vi "Calc_Remaining_Time.vi"(2 "Currently on Row":i32, 3 "Table In":T1[](array[typedef]) {"Row Duration (mins)" format="%#.1f"; "Row No" min=0; "Trace Gas Concentration (%)" min=0.0 format="%#.2f"; "Emission Rate (l/min)" format="%#.2f"; "Tunnel Speed" format="%#.2f"; "Start X" format="%#.2f"; "Start Y" format="%#.2f"; "Start Z" format="%#.2f"; "End X" format="%#.2f"; "End Y" format="%#.2f"; "End Z" format="%#.2f"; "Averaging time (min)" min=0.0 format="%#.2f"}) -> (0 "Estimated Completion time":string, 1 "Table Out":T1[](array[typedef]) {"Row Duration (mins)" format="%#.1f"; "Row No" min=0; "Trace Gas Concentration (%)" min=0.0 format="%#.2f"; "Emission Rate (l/min)" format="%#.2f"; "Tunnel Speed" format="%#.2f"; "Start X" format="%#.2f"; "Start Y" format="%#.2f"; "Start Z" format="%#.2f"; "End X" format="%#.2f"; "End Y" format="%#.2f"; "End Z" format="%#.2f"; "Averaging time (min)" min=0.0 format="%#.2f"})   [LabVIEW 2010]
uses:
  Traverse_cluster.ctl
  Spacing.ctl
  Controls/Multi_run_mode.ctl
  Controls/Overhead.ctl
  Globals/Extra_Commands_Global.vi
  Globals/Trav_pos_global.vi
panel:
  # "X           Y            Z"
  # "Start"
  # "End"
  # "X           Y            Z"
  # "Start"
  # "End"
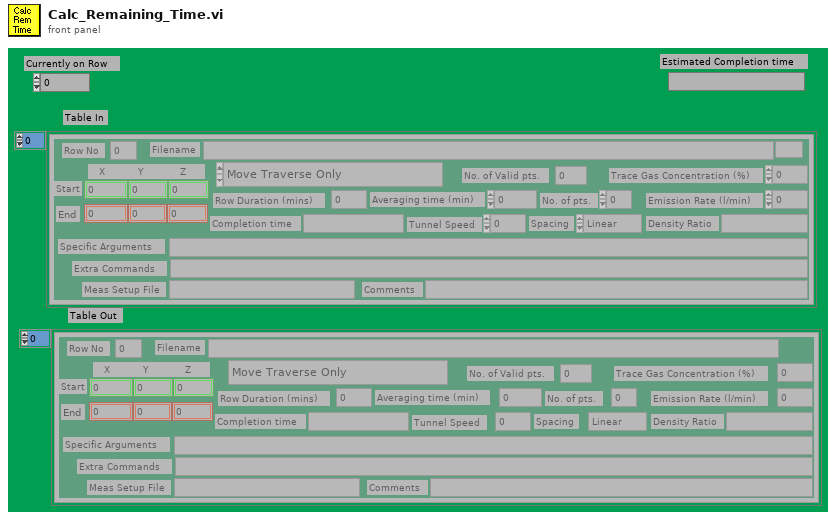
[diagram p1: front panel]
types:
  T1 = typedef "Traverse_cluster.ctl" = cluster{"Start X":dbl, "Start Y":dbl, "Start Z":dbl, "End X":dbl, "End Y":dbl, "End Z":dbl, "No. of pts.":i32, "Spacing":T2, "Filename":path, "Tunnel Speed":dbl, "Averaging time (min)":dbl, "Extra Commands":string, "Specific Arguments":string, "Emission Rate (l/min)":dbl, "Trace Gas Concentration (%)":dbl, "Density Ratio":string, "Comments":string, "Row No":i32, "Row Type Selector":T3, "Completion time":string, "Row Duration (mins)":dbl, "No. of Valid pts.":i32, "Meas Setup File":string}
  T2 = typedef "Spacing.ctl" = enum16{"Linear", "Log", "Gauss", "Specified", "N/A"}
  T3 = typedef "Multi_run_mode.ctl" = enum16{"Move Traverse Only", "Set Tunnel Speed Only", "Set Source Only", "Set Measurement Conditions", "Single Measurement", "Vertical Profile", "Lateral Profile", "Longitudinal Profile", "Explore Volume", "Multi-Axis Profile", "Auto Calibrate", "Meas Fast FID Bkgnd", "Check Beam Power", "Scanning Valve Measurement", "Run VI Named:", "Set ADAM Ch", "Wait (minutes)", "Send Message", "Synchronize With:", "Fall Back to this Row", "Turn Off Row Repeating", "Blank Row"}
  T4 = typedef "Overhead.ctl" = enum16{"Update total times", "Read Current Overhead", "Re Scale totals to 3 hrs", "Initialise totals to 3hr"}
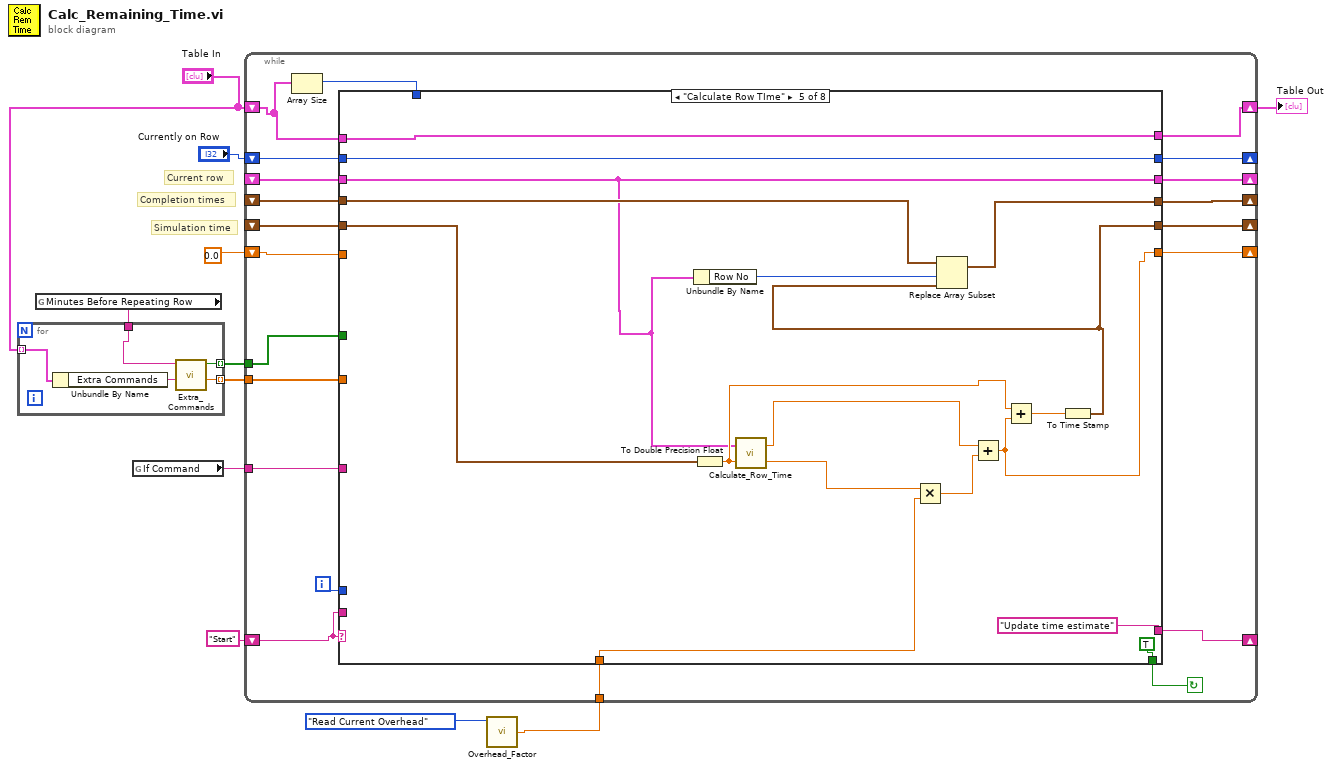
[diagram p0: block diagram]
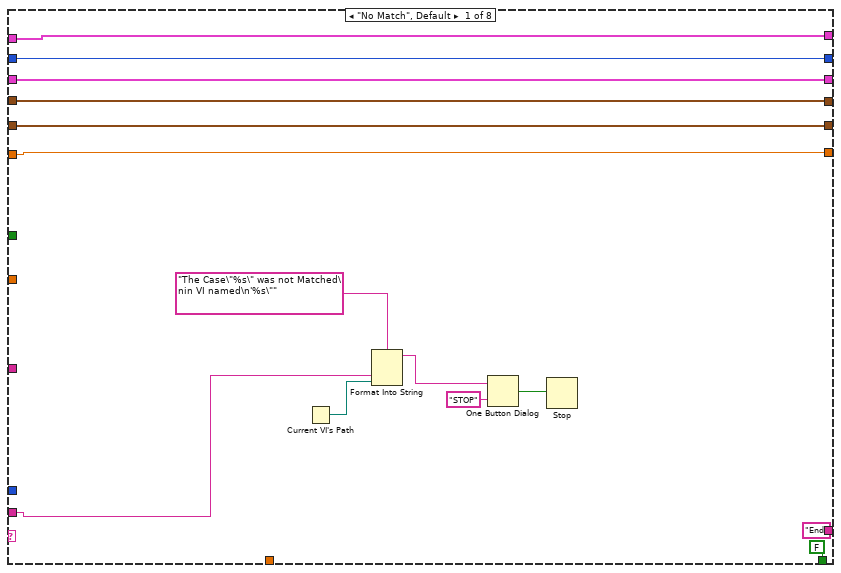
[diagram p2: hidden frame]
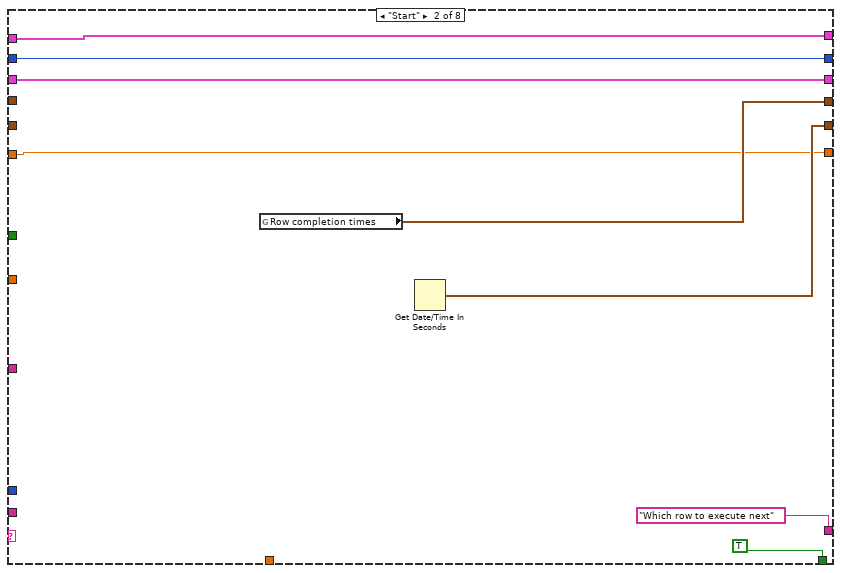
[diagram p3: hidden frame]
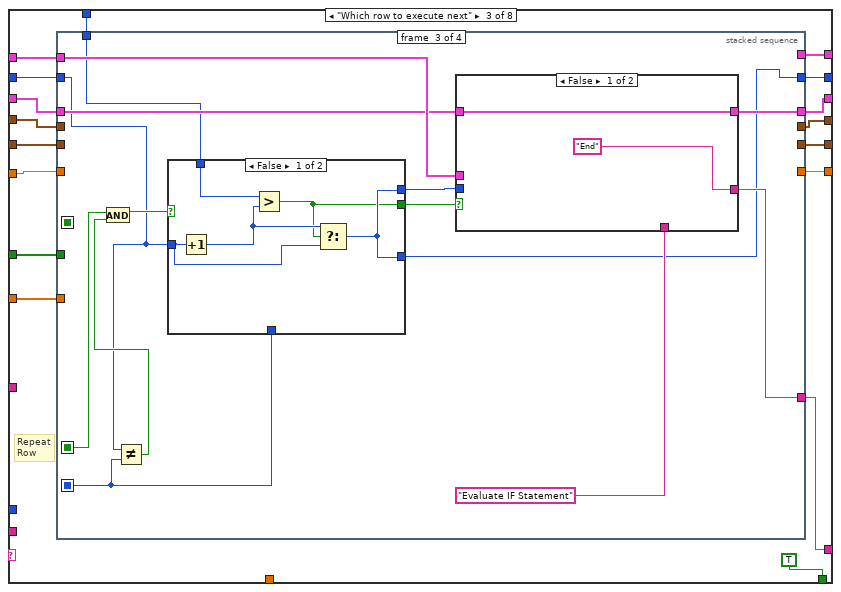
[diagram p4: hidden frame]
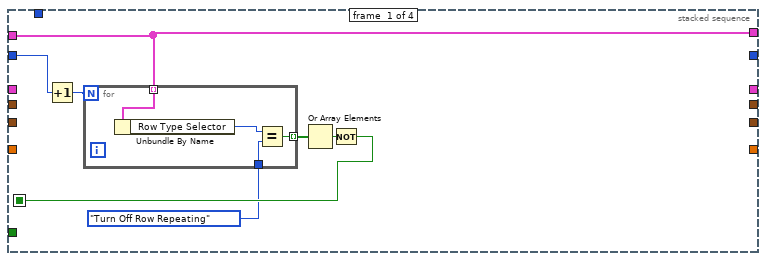
[diagram p5: hidden frame]
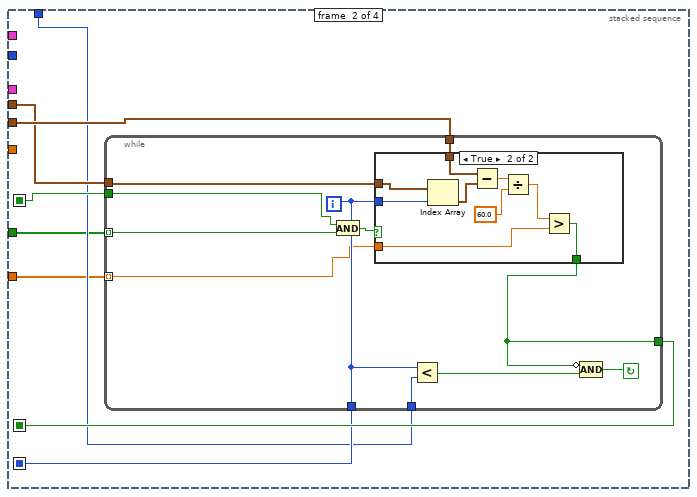
[diagram p6: hidden frame]
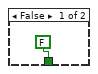
[diagram p7: hidden frame]
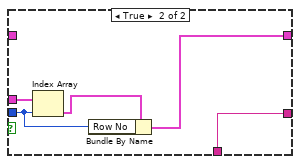
[diagram p8: hidden frame]
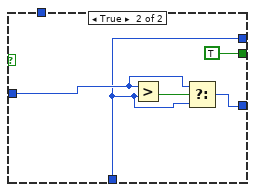
[diagram p9: hidden frame]
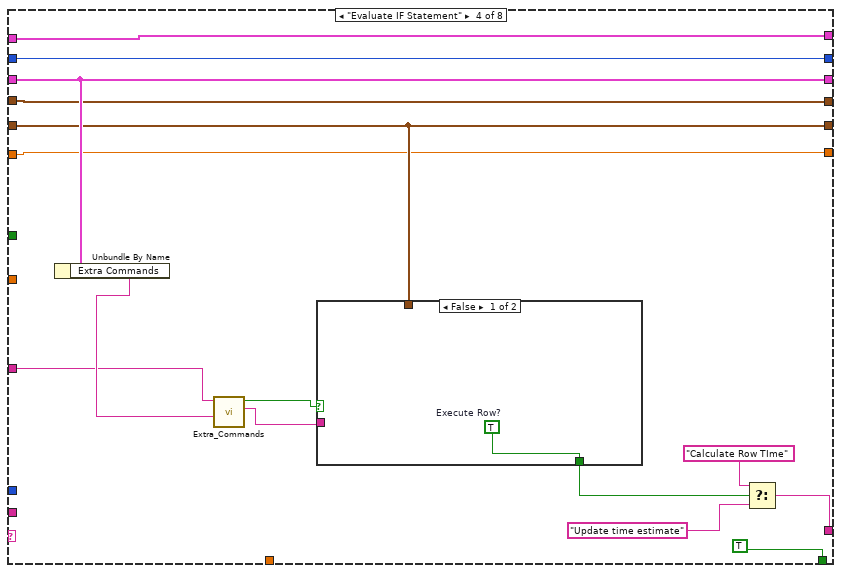
[diagram p11: hidden frame]
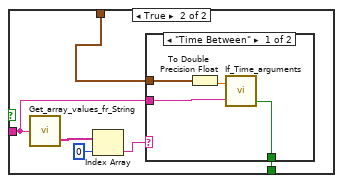
[diagram p12: hidden frame]
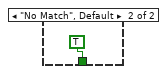
[diagram p13: hidden frame]
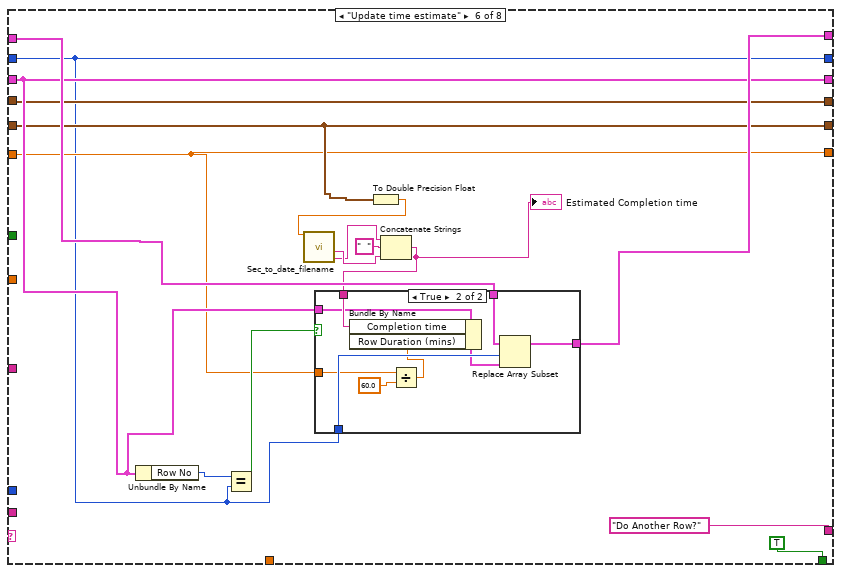
[diagram p14: hidden frame]
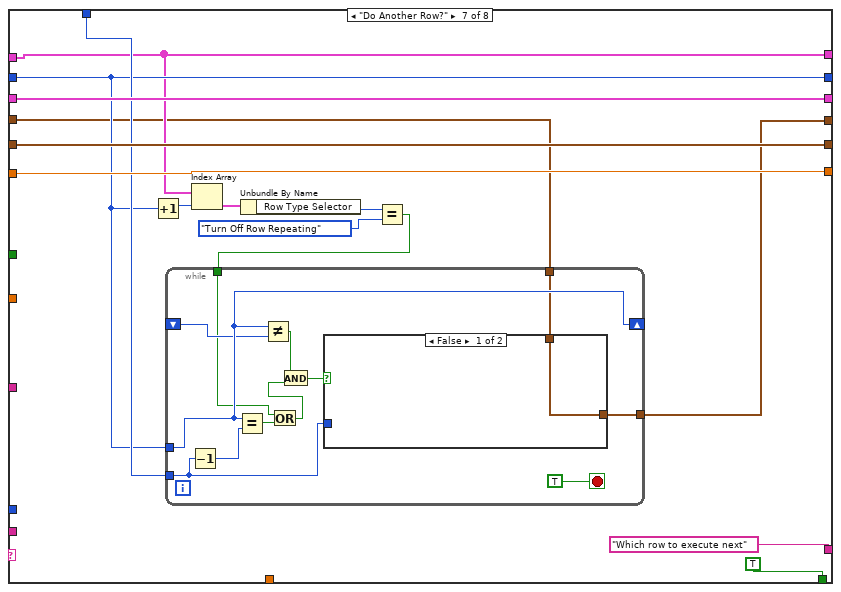
[diagram p16: hidden frame]
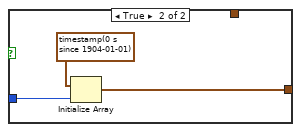
[diagram p17: hidden frame]
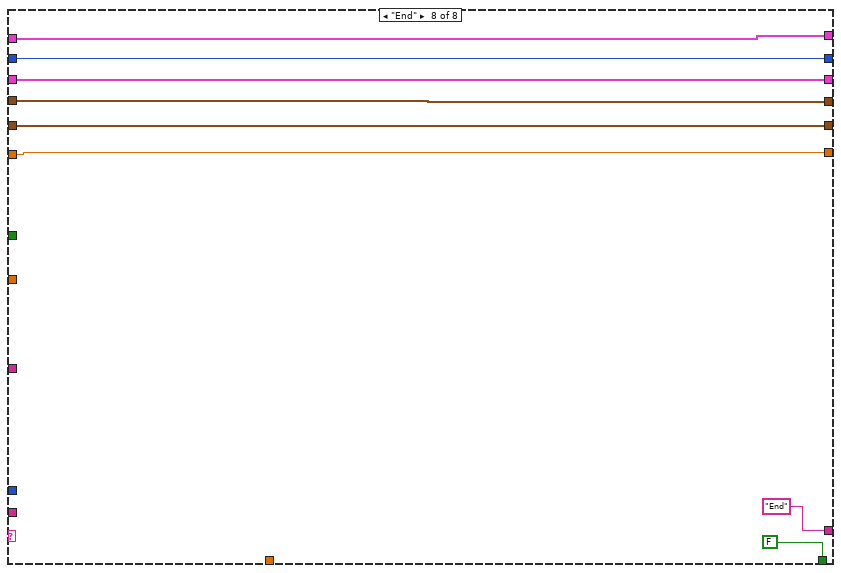
[diagram p18: hidden frame]
diagram:
  # "Simulation time"
  # "Completion times"
  # "Current row"
  n1 = global read "Extra_Commands_Global.vi" "Minutes Before Repeating Row"() -> (w1:string)
  n2 = for {
    tunnel: "Table In" -> [w15] mode=indexing
    tunnel: [w14] -> w3 mode=indexing
    tunnel: [w13] -> w2 mode=indexing
    tunnel: w1 -> [w12]
    n3 = Unbundle By Name(w15) -> ("Extra Commands"=w16:string)
    n4 = call "Extra_Commands.vi"("String to Search"=w16, "Command"=w12) -> ("Numeric Value"=w13:dbl, "Command Found"=w14:bool)  [unwired: 1 in, 3 out]
  }
  n5 = global read "Extra_Commands_Global.vi" "If Command"() -> (w7:string)
  n6 = call "Overhead_Factor.vi"("Mode"=Overhead."Read Current Overhead") -> ("Current Overhead Factor"=w8:dbl)  [unwired: 3 in]
  n7 = while {
    shift-left: "Start" -> [w35]
    shift-right: [w34] -> _
    shift-right: [w32] -> w10
    shift-left: "Table In" -> [w21]
    tunnel: w8 -> [w31]
    shift-right: [w30] -> _
    shift-left: _ -> [w29]
    shift-right: [w25] -> _
    shift-left: _ -> [w26]
    shift-right: [w27] -> _
    shift-left: _ -> [w28]
    shift-right: [w22] -> _
    shift-left: "Currently on Row" -> [w23]
    tunnel: w7 -> [w24]
    shift-right: [w20] -> _
    shift-left: 0.0 ("row Duration") -> [w19]
    tunnel: w3 -> [w18]
    tunnel: w2 -> [w17]
    i -> [w36]
    stop <- w37 continue-if-true
    n8 = Array Size(array=w21) -> (size(s)=w33:i32)
    n9 = case shown="\"Calculate Row TIme\"" w35 {
      tunnel: [FALSE ("Continue?") TRUE ("Continue?") TRUE ("Continue?") TRUE TRUE TRUE TRUE FALSE] -> w37
      tunnel: w21 -> [w45 w59 w74 w162 w193 w209 w223 w258]
      tunnel: w35 -> [w46 _ _ _ _ _ _ _]
      tunnel: w36 -> [_ _ _ _ _ _ _ _]
      tunnel: ["End" "Which row to execute next" w72 w164 "Update time estimate" "Do Another Row?" "Which row to execute next" "End"] -> w34
      tunnel: w33 -> [_ _ w73 _ _ _ w229 _]
      tunnel: [w45 w59 w75 w162 w193 w208 w223 w258] -> w32
      tunnel: w31 -> [_ _ _ _ w186 _ _ _]
      tunnel: [w42 w54 w71 w154 w180 w199 w233 w256] -> w30
      tunnel: w29 -> [w42 w54 w70 w154 w180 w199 w233 w256]
      tunnel: w28 -> [w39 _ w69 w152 w181 w197 w232 w254]
      tunnel: [w39 w56 w64 w152 w184 w197 w232 w254] -> w27
      tunnel: w26 -> [w40 _ w68 w153 w183 w198 w221 w255]
      tunnel: [w40 w55 w65 w153 w182 w198 w230 w255] -> w25
      tunnel: w24 -> [_ _ _ w156 _ _ _ _]
      tunnel: w23 -> [w41 w53 w67 w155 w179 w195 w224 w253]
      tunnel: [w41 w53 w66 w155 w179 w195 w224 w253] -> w22
      tunnel: [w38 w52 w62 w151 w178 w196 w231 w252] -> w20
      tunnel: w19 -> [w38 w52 w63 w151 _ w196 w231 w252]
      tunnel: w18 -> [_ _ w61 _ _ _ _ _]
      tunnel: w17 -> [_ _ w60 _ _ _ _ _]
      frame "No Match", Default {
        n10 = Current VI's Path() -> (path=w47:path)
        n11 = Format Into String(format string="The Case\"%s\" was not Matched\nin VI named\n'%s\"" ("Format String"), w46, w47) -> (resulting string=w50:string)  [unwired: 2 in, 1 out]
        n12 = One Button Dialog(message=w50, button name ("OK")="STOP") -> (true=w48:bool)
        n13 = Stop(stop? (T)=w48) -> ()
      }
      frame "Start" {
        n14 = global read "Trav_pos_global.vi" "Row completion times"() -> (w55:timestamp[])
        n15 = Get Date/Time In Seconds() -> (seconds since 1Jan1904=w56:timestamp)
      }
      frame "Which row to execute next" {
        # "Repeat\nRow"
        n16 = stacked-sequence {
          seq-local: [_ w95 _ _] -> [_ _ w125 _]
          seq-local: [_ w94 _ _] -> [_ _ w126 _]
          seq-local: [w80 _ _ _] -> [_ w93 _ _]
          tunnel: [w79 _ _ _] -> w75
          tunnel: w74 -> [w79 _ w129 _]
          tunnel: w73 -> [_ w90 w118 _]
          tunnel: [_ _ w127 _] -> w72
          tunnel: [_ _ w121 _] -> w71
          tunnel: w70 -> [_ _ w120 _]
          tunnel: w69 -> [_ w92 _ w149]
          tunnel: w68 -> [_ w91 _ w150]
          tunnel: w67 -> [w77 _ w119 _]
          tunnel: [_ _ w117 _] -> w66
          tunnel: [_ _ _ w150] -> w65
          tunnel: [_ _ _ w149] -> w64
          tunnel: w63 -> [_ _ _ w148]
          tunnel: [_ _ _ w148] -> w62
          tunnel: w61 -> [_ w89 _ _]
          tunnel: w60 -> [_ w88 _ _]
          frame #0 {
            n17 = Increment(x=w77) -> (x+1=w82:i32)
            n18 = for {
              N: w82 -> [_]
              tunnel: w79 -> [w87] mode=indexing
              tunnel: [w85] -> w83 mode=indexing
              tunnel: Multi_run_mode."Turn Off Row Repeating" ("Row Type Selector") -> [w84]
              n19 = Unbundle By Name(w87) -> ("Row Type Selector"=w86:T3)
              n20 = Equal?(x=w86, y=w84) -> (x = y?=w85:bool)
            }
            n21 = Or Array Elements(Boolean array=w83) -> (logical OR=w81:bool)
            n22 = Not(x=w81) -> (.not. x?=w80:bool)
          }
          frame #1 {
            n23 = while {
              tunnel: w91 -> [w106]
              tunnel: w92 -> [w105]
              tunnel: [w99] -> w95
              tunnel: [w98] -> w94
              tunnel: w93 -> [w102]
              tunnel: w90 -> [w100]
              tunnel: w89 -> [w97] mode=indexing
              tunnel: w88 -> [w96] mode=indexing
              i -> [w98]
              stop <- w104 continue-if-true
              n24 = And(x=w102, y=w97) -> (x .and. y?=w101:bool)
              n25 = case shown="True" w101 {
                tunnel: w106 -> [_ w112]
                tunnel: w105 -> [_ w113]
                tunnel: w98 -> [_ w111]
                tunnel: w96 -> [_ w109]
                tunnel: [FALSE w108] -> w99
                frame False {
                }
                frame True {
                  n26 = Index Array(array=w112, index=w111) -> (element=w114:timestamp)
                  n27 = Subtract(x=w113, y=w114) -> (x-y=w115:dbl)
                  n28 = Divide(x=w115, y=60.0) -> (x/y=w110:dbl)
                  n29 = Greater?(x=w110, y=w109) -> (0:w108:bool)
                }
              }
              n30 = Less?(x=w98, y=w100) -> (x < y?=w103:bool)
              n31 = Compound Arithmetic op=AND(invert w99, w103) -> (w104:bool)
            }
          }
          frame #2 {
            n32 = Not Equal?(x=w119, y=w126) -> (x != y?=w124:bool)
            n33 = And(x=w125, y=w124) -> (x .and. y?=w123:bool)
            n34 = case shown="False" w123 {
              tunnel: w126 -> [_ w144]
              tunnel: w119 -> [w140 w146]
              tunnel: [w139 w145] -> w117
              tunnel: [w139 w144] -> w130
              tunnel: w118 -> [w142 _]
              tunnel: [w138 TRUE] -> w128
              frame False {
                n35 = Increment(x=w140) -> (x+1=w141:i32)
                n36 = Greater?(x=w142, y=w141) -> (0:w138:bool)
                n37 = Select(t=w141, s=w138, f=w140) -> (s? t:f=w139:i32)
              }
              frame True {
                n38 = Greater?(x=w146, y=w144) -> (0:w147:bool)
                n39 = Select(t=w146, s=w147, f=w144) -> (s? t:f=w145:i32)
              }
            }
            n40 = case shown="False" w128 {
              tunnel: w130 -> [_ w134]
              tunnel: w129 -> [_ w137]
              tunnel: ["End" w136] -> w127
              tunnel: "Evaluate IF Statement" -> [_ w136]
              tunnel: [w131 w133] -> w121
              tunnel: w120 -> [w131 _]
              frame False {
              }
              frame True {
                n41 = Index Array(array=w137, index=w134) -> (element=w135:T1)
                n42 = Bundle By Name(cluster=w135, "Row No"=w134) -> (w133:T1)
              }
            }
          }
          frame #3 {
          }
        }
      }
      frame "Evaluate IF Statement" {
        n43 = Unbundle By Name(w154) -> ("Extra Commands"=w161:string)
        n44 = call "Extra_Commands.vi"("String to Search"=w161, "Command"=w156) -> ("String Value"=w163:string, "Command Found"=w159:bool)  [unwired: 1 in, 3 out]
        n45 = case shown="False" w159 {
          tunnel: w163 -> [_ w169]
          tunnel: [w166 w168] -> w160
          tunnel: w152 -> [_ w167]
          frame False {
            w166 = TRUE  # Execute Row?
          }
          frame True {
            n46 = call "Get_array_values_fr_String.vi"("String Value"=w169) -> ("String array"=w171:string[])  [unwired: 1 out]
            n47 = Index Array(array=w171, index=0 ("Index")) -> (element=w170:string)
            n48 = case shown="\"Time Between\"" w170 {
              tunnel: w169 -> [w176 _]
              tunnel: [w175 TRUE ("Execute Row?")] -> w168
              tunnel: w167 -> [w173 _]
              frame "Time Between" {
                n49 = To Double Precision Float(number=w173) -> (double precision float=w174:dbl)
                n50 = call "If_Time_arguments.vi"("seconds since 1Jan1904"=w174, "String Value"=w176) -> ("Execute Row?"=w175:bool)  [unwired: 2 out]
              }
              frame "No Match", Default {
              }
            }
          }
        }
        n51 = Select(t="Calculate Row TIme", s=w160, f="Update time estimate") -> (s? t:f=w164:string)
      }
      frame "Calculate Row TIme" {
        n52 = Unbundle By Name(w180) -> ("Row No"=w192:i32)
        n53 = To Double Precision Float(number=w181) -> (double precision float=w189:dbl)
        n54 = call "Calculate_Row_Time.vi"("Row Start Time (Sec Since 1904)"=w189, "Multi Run Row"=w180) -> ("Scalable Time (Sec)"=w187:dbl, "Fixed Time (Sec)"=w190:dbl)
        n55 = Multiply(x=w187, y=w186) -> (x*y=w191:dbl)
        n56 = Add(x=w190, y=w191) -> (x+y=w178:dbl)
        n57 = Add(x=w189, y=w178) -> (x+y=w188:dbl)
        n58 = To Time Stamp(1:w188) -> (0:w184:timestamp)
        n59 = Replace Array Subset(array=w183, new element=w184, index=w192) -> (w182:timestamp[])
      }
      frame "Update time estimate" {
        n60 = Unbundle By Name(w199) -> ("Row No"=w207:i32)
        n61 = Equal?(x=w207, y=w195) -> (x = y?=w206:bool)
        n62 = To Double Precision Float(number=w197) -> (double precision float=w202:dbl)
        n63 = call "Sec_to_date_filename.vi"("seconds"=w202) -> ("Day"=w204:string, "Time"=w203:string)  [unwired: 2 out]
        n64 = Concatenate Strings(w203, "  " ("Substring"), w204) -> (w201:string)
        "Estimated Completion time" <- w201
        n65 = case shown="True" w206 {
          tunnel: w195 -> [_ w220]
          tunnel: w209 -> [w211 w219]
          tunnel: [w211 w217] -> w208
          tunnel: w201 -> [_ w216]
          tunnel: w199 -> [_ w215]
          tunnel: w196 -> [_ w212]
          frame False {
          }
          frame True {
            n66 = Divide(x=w212, y=60.0) -> (x/y=w213:dbl)
            n67 = Bundle By Name(cluster=w215, "Completion time"=w216, "Row Duration (mins)"=w213) -> (w218:T1)
            n68 = Replace Array Subset(array=w219, new element=w218, index=w220) -> (w217:T1[])
          }
        }
      }
      frame "Do Another Row?" {
        n69 = Increment(x=w224) -> (x+1=w227:i32)
        n70 = Index Array(array=w223, index=w227) -> (element=w228:T1)
        n71 = Unbundle By Name(w228) -> ("Row Type Selector"=w225:T3)
        n72 = Equal?(x=w225, y=Multi_run_mode."Turn Off Row Repeating" ("Row Type Selector")) -> (x = y?=w222:bool)
        n73 = while {
          shift-right: [w246] -> _
          shift-left: _ -> [w245]
          tunnel: w229 -> [w242]
          tunnel: w224 -> [w246]
          tunnel: w222 -> [w239]
          tunnel: [w237] -> w230
          tunnel: w221 -> [w236]
          stop <- TRUE stop-if-true
          n74 = Decrement(x=w242) -> (x-1=w247:i32)
          n75 = Equal?(x=w246, y=w247) -> (x = y?=w240:bool)
          n76 = Not Equal?(x=w246, y=w245) -> (x != y?=w244:bool)
          n77 = Or(x=w239, y=w240) -> (x .or. y?=w238:bool)
          n78 = And(x=w244, y=w238) -> (x .and. y?=w243:bool)
          n79 = case shown="False" w243 {
            tunnel: w242 -> [_ w250]
            tunnel: [w248 w249] -> w237
            tunnel: w236 -> [w248 _]
            frame False {
            }
            frame True {
              n80 = Initialize Array(timestamp(0 s since 1904-01-01) ("seconds since 1Jan1904"), w250) -> (w249:timestamp[])
            }
          }
        }
      }
      frame "End" {
      }
    }
  }
  "Table Out" <- w10
